vi "TSCAN_DBWrite.vi"(8 "错误输入（无错误）":errorcluster, 9 "AId":i32 format="%x", 10 "簇":T1, 11 "路径输入":path) -> (0 "错误输出":errorcluster, 3 "路径输出":path)   [LabVIEW 2019]
panel:
  in  "AIsData":u8(ring) items=["数据帧", "远程帧"]
  in  "AIsStd":u8(ring) items=["标准帧", "扩展帧"]
  in  "FIdxChn":u8
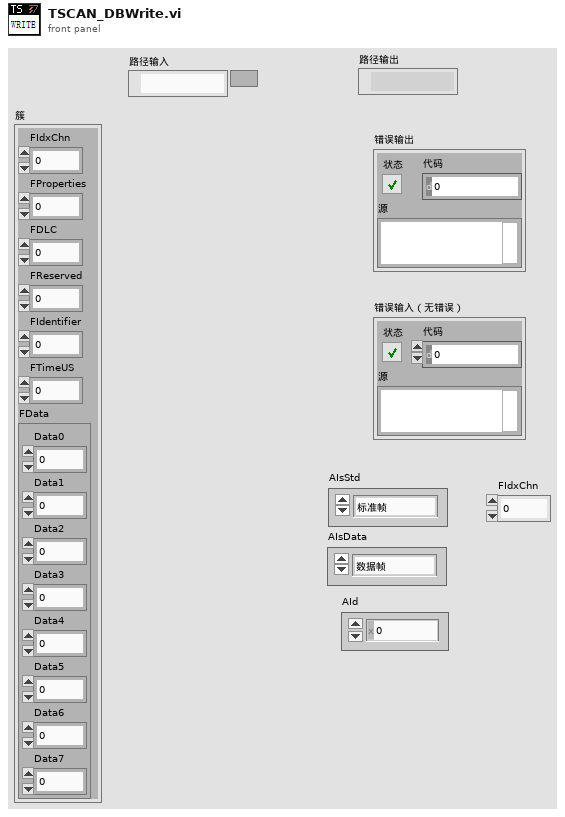
[diagram p1: front panel]
types:
  T1 = cluster{"FIdxChn":u8, "FProperties":u8, "FDLC":u8, "FReserved":u8, "FIdentifier":i32, "FTimeUS":u64, "FData":cluster{"Data0":u8, "Data1":u8, "Data2":u8, "Data3":u8, "Data4":u8, "Data5":u8, "Data6":u8, "Data7":u8}}
  T2 = cluster{"Data0":u8, "Data1":u8, "Data2":u8, "Data3":u8, "Data4":u8, "Data5":u8, "Data6":u8, "Data7":u8}
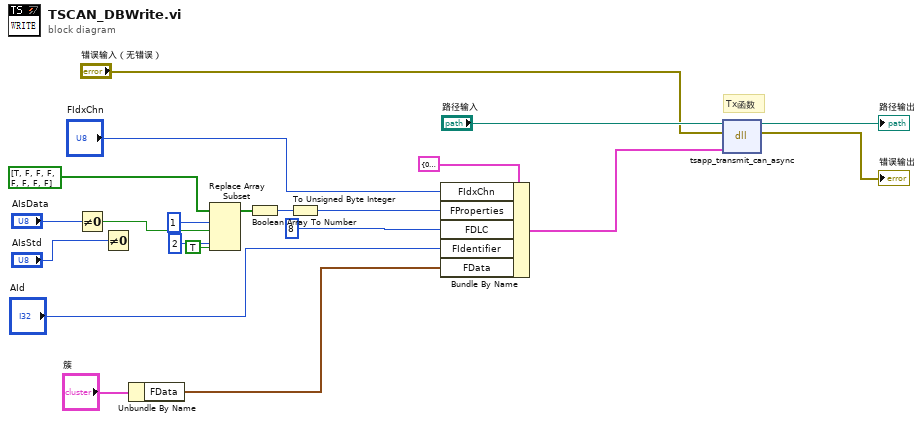
[diagram p0: block diagram]
diagram:
  # "Tx函数"
  n1 = Not Equal To 0?(x="AIsData") -> (x != 0?=w11:bool)
  n2 = Not Equal To 0?(x="AIsStd") -> ()  [unwired: 1 out]
  n3 = Unbundle By Name("簇") -> ("FData"=w14:T2)
  n4 = Replace Array Subset(array=bool[] [TRUE, FALSE, FALSE, FALSE, FALSE, FALSE, FALSE, FALSE], new element #1=w11, index #1=1 ("索引"), new element #2=TRUE ("新元素/子数组"), index #2=2 ("索引")) -> (w8:bool[])
  n5 = Boolean Array To Number(Boolean array=w8) -> (number=w7:u32)
  n6 = To Unsigned Byte Integer(number=w7) -> (unsigned 8bit integer=w6:u8)
  n7 = Bundle By Name(cluster=T1 {"FIdxChn"=0, "FProperties"=0, "FDLC"=0, "FReserved"=0, "FIdentifier"=0, "FTimeUS"=0, "FData"={"Data0"=0, "Data1"=0, "Data2"=0, "Data3"=0, "Data4"=0, "Data5"=0, "Data6"=0, "Data7"=0}} ("簇"), "FIdxChn"="FIdxChn", "FProperties"=w6, "FDLC"=u8 8, "FIdentifier"="AId", "FData"=w14) -> (w16:T1)
  n8 = dll-call lib="C:/Users/Administrator/Desktop/TS_Can/Path/TSMaster.dll" fn="tsapp_transmit_can_async"(path in="路径输入", error in="错误输入（无错误）", "ACAN"=w16) -> (path out=→"路径输出":path, error out=→"错误输出":errorcluster)  [unwired: 3 in]
